vi "InitSV.vi"(8 "error in (no error)":errorcluster, 9 "PowerSV refnum":refnum<k21>, 10 "TriggerSV refnum":refnum<k21>, 11 "UniStableShutter in":refnum<class "UniStableShutter.lvclass">) -> (0 "error out":errorcluster, 3 "UniStableShutter out":refnum<class "UniStableShutter.lvclass">)   [LabVIEW 2016, in "UniStableShutter.lvclass"]
uses:
  UniStableShutter.lvclass
  UniStableShutter.lvclass/UniStableShutter.ctl
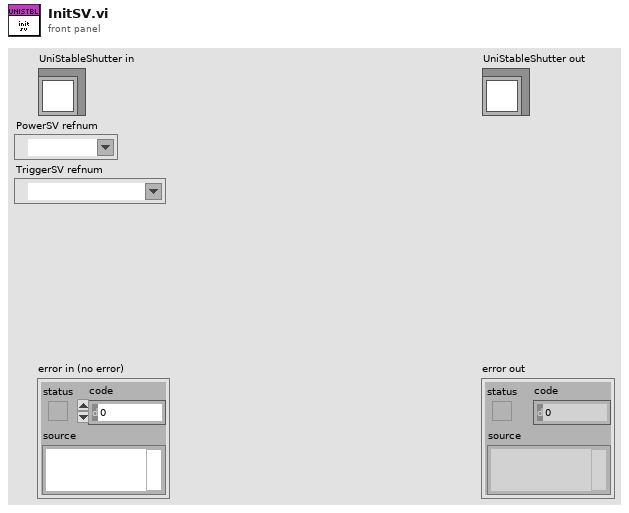
[diagram p1: front panel]
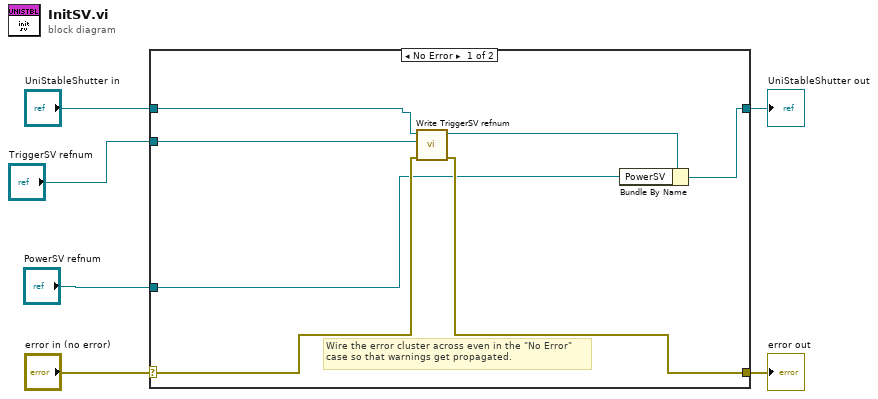
[diagram p0: block diagram]
diagram:
  n1 = case shown="No Error" "error in (no error)" {
    selector: "error in (no error)" -> [w10 w15]
    tunnel: [w9 w15] -> w5
    tunnel: [w13 w14] -> w3
    tunnel: "UniStableShutter in" -> [w12 w14]
    tunnel: "TriggerSV refnum" -> [w11 _]
    tunnel: "PowerSV refnum" -> [w7 _]
    frame No Error {
      # "Wire the error cluster across even in the \"No Error\"\ncase so that warnings get propagated."
      n2 = call-dynamic "Write TriggerSV refnum.vi"("error in (no error)"=w10, "TriggerSV refnum"=w11, "Shutter in"=w12) -> ("error out"=w9:errorcluster, "Shutter out"=w8:refnum<class "UniStableShutter.lvclass">)  [unwired: 7 in]
      n3 = Bundle By Name(cluster=w8, "PowerSV"=w7) -> (w13:refnum<class "UniStableShutter.lvclass">)
    }
    frame Error {
    }
  }
  "error out" <- w5
  "UniStableShutter out" <- w3
